vi "VI-Replace Event Data in Events.vi"(7 "Events typedef":path, 11 "error in (no error)":errorcluster, 12 "Event Data typedef":path) -> (15 "error out":errorcluster)   [LabVIEW 2015]
uses:
  <vilib>/Utility/traverseref.llb/TRef TravTarget.ctl
  <vilib>/Utility/miscctls.llb/LVPositionTypeDef.ctl
  <vilib>/Utility/traverseref.llb/VI Scripting - Traverse.lvlib
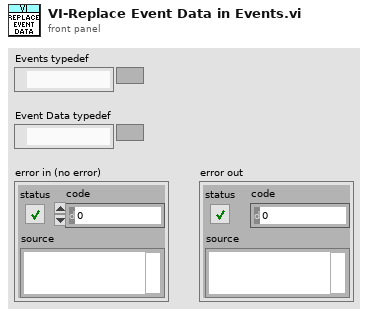
[diagram p1: front panel]
types:
  T1 = typedef "LVPositionTypeDef.ctl" = cluster{"Left":i32, "Top":i32}
  T2 = typedef "TRef TravTarget.ctl" = enum16{"FP", "BD", "Other"}
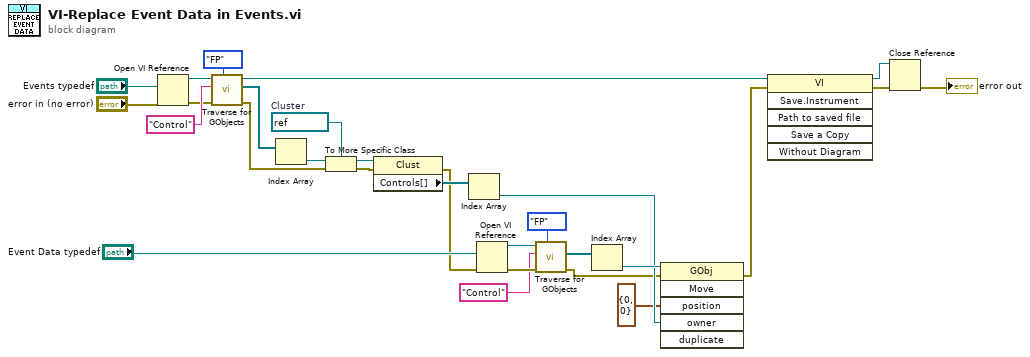
[diagram p0: block diagram]
diagram:
  w19 = refnum<vi> refnum  # Cluster
  n1 = Open VI Reference(vi path="Events typedef", error in (no error)="error in (no error)") -> (vi reference=w23:refnum<vi>, error out=w14:errorcluster)  [unwired: 4 in]
  n2 = call <vilib>:"Traverse for GObjects.vi"("Traverse Target"=TRef_TravTarget."FP", "error in (no error)"=w14, "Class Name"="Control", "VI Refnum"=w23) -> ("error out"=w16:errorcluster, "References"=w20:refnum<vi>[], "dup VI Refnum"=w25:refnum<vi>)  [unwired: 4 in, 1 out]
  n3 = Index Array(array=w20) -> (element=w13:refnum<vi>)  [unwired: 1 in]
  n4 = To More Specific Class(target class=w19, reference=w13, error in=w16) -> (specific class reference=w17:refnum<vi>, error out=w18:errorcluster)
  n5 = property class="Clust"(reference=w17, error in=w18) -> (error out=w2:errorcluster, "Controls[]"=w24:refnum<vi>[])  [unwired: 1 out]
  n6 = Index Array(array=w24) -> (element=w5:refnum<vi>)  [unwired: 1 in]
  n7 = Open VI Reference(vi path="Event Data typedef", error in (no error)=w2) -> (vi reference=w10:refnum<vi>, error out=w9:errorcluster)  [unwired: 4 in]
  n8 = call <vilib>:"Traverse for GObjects.vi"("Traverse Target"=TRef_TravTarget."FP", "error in (no error)"=w9, "Class Name"="Control", "VI Refnum"=w10) -> ("error out"=w1:errorcluster, "References"=w7:refnum<vi>[])  [unwired: 4 in, 2 out]
  n9 = Index Array(array=w7) -> (element=w6:refnum<vi>)  [unwired: 1 in]
  n10 = invoke class="GObj" method="Move"(reference=w6, error in=w1, "position"=T1 {"Left"=0, "Top"=0}, "owner"=w5) -> (error out=w3:errorcluster)  [unwired: 2 in, 5 out]
  n11 = invoke class="VI" method="Save.Instrument"(reference=w25, error in=w3) -> (reference out=w27:refnum<vi>, error out=w26:errorcluster)  [unwired: 4 in, 4 out]
  n12 = Close Reference(reference=w27, error in (no error)=w26) -> (error out=→"error out":errorcluster)
